vi "Swerve Drive.vi"(0 "X":dbl(slide) scale=-1.0..1.0, 1 "Rot. Point Y":dbl, 3 "Rot. Point X":dbl, 7 "Y":dbl(slide) scale=1.0..-1.0, 11 "Z":dbl(knob) scale=1.0..-1.0, 13 "Robot-Centric":bool) -> ()   [LabVIEW 2018]
panel:
  out "YAW":dbl format="%#_13g"
  in  "Robot Length":dbl=21.5
  in  "Robot Width":dbl=29.5
  # "SWERVE DRIVE\nVersion 3.1B\n\nCory Lynch\nApple Pi Robotics\nTeam 2067\n\nAdapted by\nDavid Genois\nfor Team 5443"
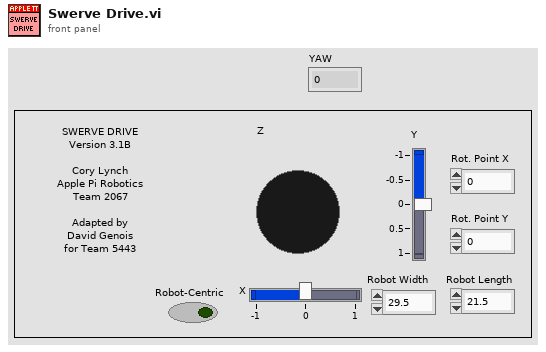
[diagram p1: front panel]
types:
  T1 = enum16{"Back Left", "Back Right", "Front Left", "Front Right"}
  T2 = typedef "WPI_GyroDevRef.ctl" = cluster{"DevStatus":errorcluster, "Analog Channel":T3, "Gain (VoltsPerDegree/Second)":dbl, "Gyro Type":enum16{"Analog", "XRS450"}, "Handle":i32, "SPI Bus":T4, "Device Found":bool, "Sample Rate":dbl, "Calibrate On Open":bool, "Offset":dbl}
  T3 = typedef "FPGA_AIChannel.ctl" = enum8{"AI 0", "AI 1", "AI 2", "AI 3", "AI MXP 0", "AI MXP 1", "AI MXP 2", "AI MXP 3", "Invalid"}
  T4 = typedef "spi_bus.ctl" = enum16{"SPI On-Board, CS0", "SPI On-Board, CS1", "SPI On-Board, CS2", "SPI On-Board, CS3", "SPI MXP", "Invalid"}
  T5 = typedef "WPI_MotorControlDeviceRef.ctl" = cluster{"DeviceStatus":errorcluster, "Type":T6, "PWM":cluster{"PWM Channel":T7, "DeadBand":T8}, "CAN":cluster{"Device Number":u8, "SetOutput VI Ref":variant, "GetOutput VI Ref":variant, "Enable VI Ref":variant, "Disable VI Ref":variant, "Data":variant}, "Invert":bool, "DIO PWM":cluster{"PWM \"Enable\" Channel":T7, "DIOChannel":T9, "PWM Rate":dbl}}
  T6 = typedef "WPI_MotorControlType.ctl" = enum16{"PWM", "CAN", "DIO PWM"}
  T7 = typedef "FPGA_DIOPWMChannel.ctl" = enum8{"PWM 0", "PWM 1", "PWM 2", "PWM 3", "PWM 4", "PWM 5", "PWM 6", "PWM 7", "PWM 8", "PWM 9", "PWM MXP 0", "PWM MXP 1", "PWM MXP 2", "PWM MXP 3", "PWM MXP 4", "PWM MXP 5", "PWM MXP 6", "PWM MXP 7", "PWM MXP 8", "PWM MXP 9", "Invalid"}
  T8 = typedef "WPI_PWMDeadband.ctl" = cluster{"Name":string, "maxPositivePwm":i32, "minPositivePwm":i32, "centerPwm":i32, "maxNegativePwm":i32, "minNegativePwm":i32, "angularRange":u16}
  T9 = typedef "FPGA_DIOChannel.ctl" = enum8{"DIO 0", "DIO 1", "DIO 2", "DIO 3", "DIO 4", "DIO 5", "DIO 6", "DIO 7", "DIO 8", "DIO 9", "DIO MXP 0", "DIO MXP 1", "DIO MXP 2", "DIO MXP 3", "DIO MXP 4", "DIO MXP 5", "DIO MXP 6", "DIO MXP 7", "DIO MXP 8", "DIO MXP 9", "DIO MXP 10", "DIO MXP 11", "DIO MXP 12", "DIO MXP 13", "DIO MXP 14", "DIO MXP 15", "SPI Port CS1", "SPI Port CS2", "SPI Port CS3", "SPI Port MISO", "SPI Port MOSI", "Invalid"}
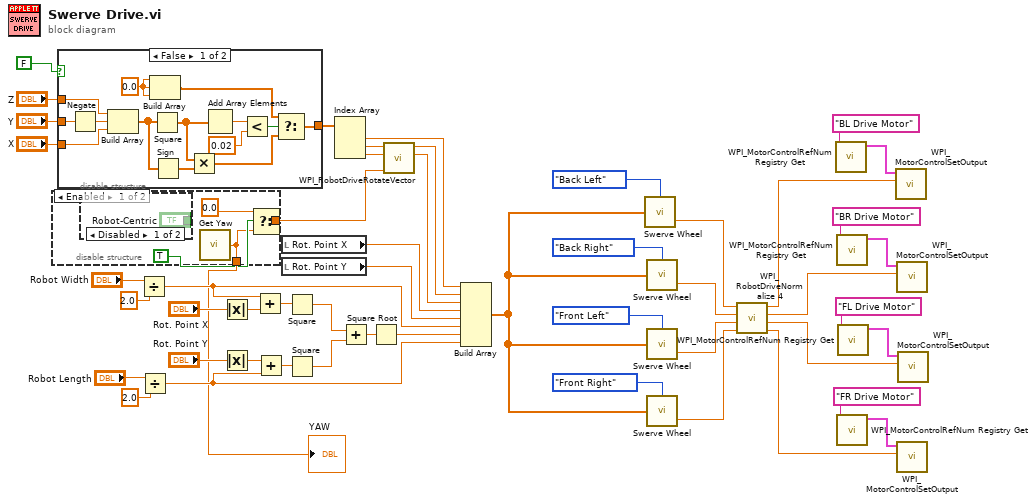
[diagram p0: block diagram]
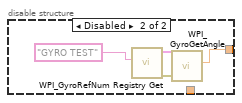
[diagram p3: hidden frame]
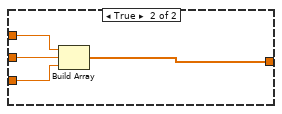
[diagram p4: hidden frame]
diagram:
  n1 = disable-structure shown="Enabled" {
    disable-tunnel: [w54 w60] -> w5
    disable-tunnel: [w52 _] -> w1
    frame Enabled {
      n2 = disable-structure shown="Disabled" {
        disable-tunnel: ["Robot-Centric" _] -> _
        frame Disabled {
        }
        frame Enabled {
        }
      }
      n3 = call "Get Yaw.vi"() -> ("Angle"=w52:dbl)  [unwired: 1 in]
      n4 = Select(t=0.0, s=TRUE, f=w52) -> (s? t:f=w54:dbl)
    }
    frame Disabled {
      n5 = call <vilib>:"WPI_GyroRefNum Registry Get.vi"("refnum name"="GYRO TEST") -> ("error out"=w59:errorcluster, "GyroDevRef"=w58:T2)  [unwired: 9 in]
      n6 = call <vilib>:"WPI_GyroGetAngle.vi"("error in"=w59, "GyroDevRef"=w58) -> ("Angle"=w60:dbl)  [unwired: 5 in, 4 out]
    }
  }
  "YAW" <- w1
  n7 = case shown="False" FALSE {
    tunnel: "Y" -> [w71 w77]
    tunnel: "X" -> [w65 w78]
    tunnel: "Z" -> [w61 w75]
    tunnel: [w62 w76] -> w8
    frame False {
      w69 = 0.0 ("element")
      n8 = Negate(x=w71) -> (-x=w64:dbl)
      n9 = Build Array(w61, w64, w65) -> (w68:dbl[])
      n10 = Build Array(w69, w69, w69) -> (w70:dbl[])
      n11 = Square(x=w68) -> (x^2=w66:dbl[])
      n12 = Sign(1:w68) -> (0:w67:dbl[])
      n13 = Multiply(x=w66, y=w67) -> (x*y=w63:dbl[])
      n14 = Add Array Elements(numeric array=w66) -> (sum=w74:dbl)
      n15 = Less?(x=w74, y=0.02 ("x")) -> (x < y?=w72:bool)
      n16 = Select(t=w70, s=w72, f=w63) -> (s? t:f=w62:dbl[])
    }
    frame True {
      n17 = Build Array(w75, w77, w78) -> (w76:dbl[])
    }
  }
  n18 = Divide(x="Robot Width", y=2.0) -> (x/y=w12:dbl)
  n19 = Divide(x="Robot Length", y=2.0) -> (x/y=w10:dbl)
  n20 = Absolute Value(x="Rot. Point X") -> (abs(x)=w30:dbl)
  n21 = Absolute Value(x="Rot. Point Y") -> (abs(x)=w28:dbl)
  n22 = Add(x=w12, y=w30) -> (x+y=w29:dbl)
  n23 = Add(x=w28, y=w10) -> (x+y=w27:dbl)
  n24 = local read "Rot. Point X"() -> (w14:dbl)
  n25 = local read "Rot. Point Y"() -> (w13:dbl)
  n26 = Square(x=w29) -> (x^2=w25:dbl)
  n27 = Square(x=w27) -> (x^2=w26:dbl)
  n28 = Index Array(array=w8) -> (element #1=w4:dbl, element #2=w9:dbl, element #3=w17:dbl)  [unwired: 3 in]
  n29 = Add(x=w25, y=w26) -> (x+y=w24:dbl)
  n30 = Square Root(x=w24) -> (sqrt(x)=w11:dbl)
  n31 = call <vilib>:"WPI_RobotDriveRotateVector.vi"("Angle"=w5, "X"=w17, "Y"=w9) -> ("X'"=w6:dbl, "Y'"=w3:dbl)  [unwired: 7 out]
  n32 = Build Array(w4, w3, w6, w14, w13, w12, w11, w10) -> (w7:dbl[])
  n33 = call "Swerve Wheel.vi"("Wheel"=T1."Back Left", "Inputs"=w7) -> ("Speed"=w48:dbl)  [unwired: 3 in]
  n34 = call "Swerve Wheel.vi"("Wheel"=T1."Back Right", "Inputs"=w7) -> ("Speed"=w47:dbl)  [unwired: 3 in]
  n35 = call "Swerve Wheel.vi"("Wheel"=T1."Front Left", "Inputs"=w7) -> ("Speed"=w46:dbl)  [unwired: 3 in]
  n36 = call "Swerve Wheel.vi"("Wheel"=T1."Front Right", "Inputs"=w7) -> ("Speed"=w45:dbl)  [unwired: 3 in]
  n37 = call <vilib>:"WPI_RobotDriveNormalize 4.vi"("D"=w45, "C"=w46, "B"=w47, "A"=w48) -> ("D'"=w32:dbl, "C'"=w33:dbl, "B'"=w34:dbl, "A'"=w35:dbl)
  n38 = call <vilib>:"WPI_MotorControlRefNum Registry Get.vi"("refnum name"="BL Drive Motor") -> ("MotorControlDevRef"=w43:T5)  [unwired: 9 in, 1 out]
  n39 = call <vilib>:"WPI_MotorControlRefNum Registry Get.vi"("refnum name"="BR Drive Motor") -> ("MotorControlDevRef"=w40:T5)  [unwired: 9 in, 1 out]
  n40 = call <vilib>:"WPI_MotorControlRefNum Registry Get.vi"("refnum name"="FR Drive Motor") -> ("MotorControlDevRef"=w36:T5)  [unwired: 9 in, 1 out]
  n41 = call <vilib>:"WPI_MotorControlRefNum Registry Get.vi"("refnum name"="FL Drive Motor") -> ("MotorControlDevRef"=w39:T5)  [unwired: 9 in, 1 out]
  n42 = call <vilib>:"WPI_MotorControlSetOutput.vi"("Output"=w35, "MotorControlDevRef"=w43) -> ()  [unwired: 7 in, 3 out]
  n43 = call <vilib>:"WPI_MotorControlSetOutput.vi"("Output"=w34, "MotorControlDevRef"=w40) -> ()  [unwired: 7 in, 3 out]
  n44 = call <vilib>:"WPI_MotorControlSetOutput.vi"("Output"=w32, "MotorControlDevRef"=w36) -> ()  [unwired: 7 in, 3 out]
  n45 = call <vilib>:"WPI_MotorControlSetOutput.vi"("Output"=w33, "MotorControlDevRef"=w39) -> ()  [unwired: 7 in, 3 out]
